vi "IECal-Create Queue Data.vi"(0 "state":T5, 7 "Params":T4) -> (8 "queue data":T1, 15 "error out":errorcluster)   [LabVIEW 2020]
uses:
  Typedefs/IECal-State.ctl
  Common VIs/Typedefs/CAL-Endpoint.ctl
  Typedefs/IECal-Parameters.ctl
  Common VIs/Typedefs/CAL-Stimulus.ctl
  Typedefs/IECal-Queue Data.ctl
  Typedefs/IECal-Response.ctl
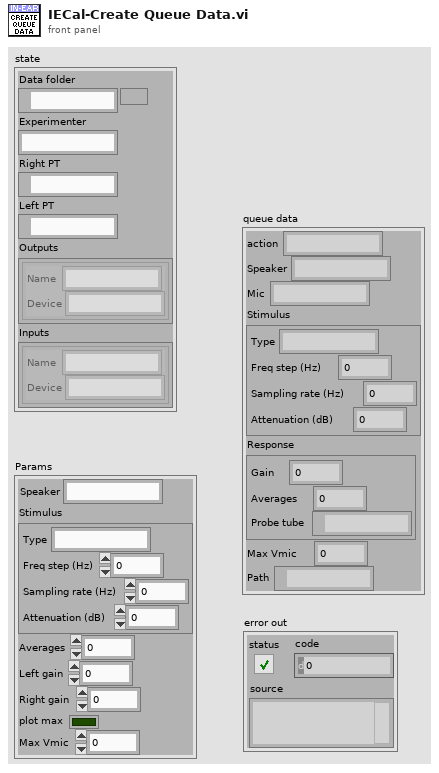
[diagram p1: front panel]
types:
  T1 = typedef "IECal-Queue Data.ctl" = cluster{"action":string, "Speaker":string, "Mic":string, "Stimulus":T2, "Response":T3, "Max Vmic":dbl, "Path":path}
  T2 = typedef "CAL-Stimulus.ctl" = cluster{"Type":string, "Freq step (Hz)":dbl, "Sampling rate (Hz)":dbl, "Attenuation (dB)":dbl}
  T3 = typedef "IECal-Response.ctl" = cluster{"Gain":dbl, "Averages":i32, "Probe tube":path}
  T4 = typedef "IECal-Parameters.ctl" = cluster{"Speaker":string, "Stimulus":T2, "Averages":i32, "Left gain":dbl, "Right gain":dbl, "plot max":bool, "Max Vmic":dbl}
  T5 = typedef "IECal-State.ctl" = cluster{"Data folder":path, "Experimenter":string, "Right PT":path, "Left PT":path, "Outputs":T6[], "Inputs":T6[]}
  T6 = typedef "CAL-Endpoint.ctl" = cluster{"Name":string, "Device":string}
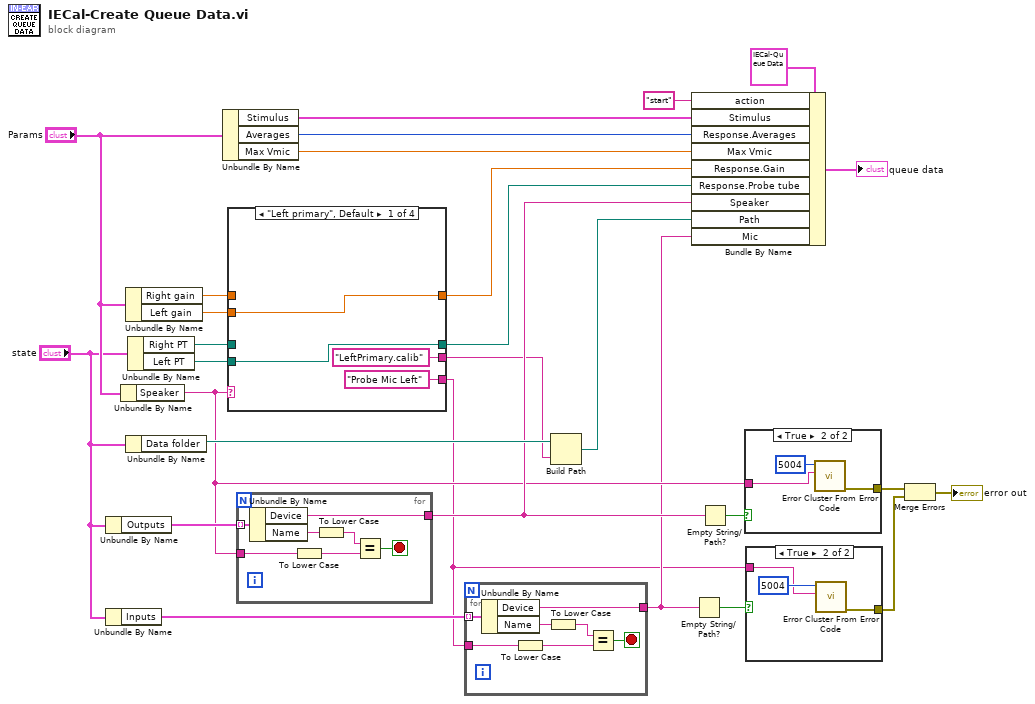
[diagram p0: block diagram]
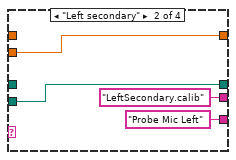
[diagram p4: hidden frame]
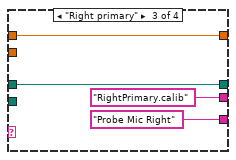
[diagram p5: hidden frame]
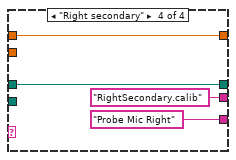
[diagram p6: hidden frame]
diagram:
  n1 = Unbundle By Name("state") -> ("Outputs"=w14:T6[])
  n2 = Unbundle By Name("state") -> ("Inputs"=w12:T6[])
  n3 = Unbundle By Name("Params") -> ("Speaker"=w9:string)
  n4 = Unbundle By Name("Params") -> ("Right gain"=w28:dbl, "Left gain"=w27:dbl)
  n5 = Unbundle By Name("state") -> ("Data folder"=w22:path)
  n6 = Unbundle By Name("state") -> ("Right PT"=w24:path, "Left PT"=w23:path)
  n7 = Unbundle By Name("Params") -> ("Stimulus"=w21:T2, "Averages"=w19:i32, "Max Vmic"=w17:dbl)
  n8 = case shown="\"Left primary\", Default" w9 {
    tunnel: w28 -> [_ _ w40 w44]
    tunnel: w27 -> [w32 w36 _ _]
    tunnel: [w32 w36 w40 w44] -> w16
    tunnel: w24 -> [_ _ w39 w43]
    tunnel: w23 -> [w31 w35 _ _]
    tunnel: [w31 w35 w39 w43] -> w15
    tunnel: ["Probe Mic Left" "Probe Mic Left" "Probe Mic Right" "Probe Mic Right"] -> w6
    tunnel: ["LeftPrimary.calib" "LeftSecondary.calib" "RightPrimary.calib" "RightSecondary.calib"] -> w2
    frame "Left primary", Default {
    }
    frame "Left secondary" {
    }
    frame "Right primary" {
    }
    frame "Right secondary" {
    }
  }
  n9 = for {
    tunnel: w14 -> [w51] mode=indexing
    tunnel: [w48] -> w11
    tunnel: w9 -> [w47]
    stop <- w49 stop-if-true
    n10 = Unbundle By Name(w51) -> ("Device"=w48:string, "Name"=w50:string)
    n11 = To Lower Case(string=w47) -> (all lower case string=w45:string)
    n12 = To Lower Case(string=w50) -> (all lower case string=w46:string)
    n13 = Equal?(x=w46, y=w45) -> (x = y?=w49:bool)
  }
  n14 = for {
    tunnel: w12 -> [w58] mode=indexing
    tunnel: [w55] -> w8
    tunnel: w6 -> [w54]
    stop <- w56 stop-if-true
    n15 = Unbundle By Name(w58) -> ("Device"=w55:string, "Name"=w57:string)
    n16 = To Lower Case(string=w54) -> (all lower case string=w52:string)
    n17 = To Lower Case(string=w57) -> (all lower case string=w53:string)
    n18 = Equal?(x=w53, y=w52) -> (x = y?=w56:bool)
  }
  n19 = Build Path(base path=w22, name or relative path=w2) -> (appended path=w1:path)
  n20 = Bundle By Name(cluster=T1 {"action"="", "Speaker"="", "Mic"="", "Stimulus"={"Type"="", "Freq step (Hz)"=0.0, "Sampling rate (Hz)"=0.0, "Attenuation (dB)"=0.0}, "Response"={"Gain"=0.0, "Averages"=0, "Probe tube"=path ""}, "Max Vmic"=0.0, "Path"=path ""} ("queue data"), "action"="start", "Stimulus"=w21, "Response.Averages"=w19, "Max Vmic"=w17, "Response.Gain"=w16, "Response.Probe tube"=w15, "Speaker"=w11, "Path"=w1, "Mic"=w8) -> (→"queue data":T1)
  n21 = Empty String/Path?(string/path=w8) -> (empty?=w7:bool)
  n22 = Empty String/Path?(string/path=w11) -> (empty?=w10:bool)
  n23 = case shown="True" w10 {
    tunnel: w9 -> [_ w60]
    tunnel: [_ w59] -> w5
    frame False {
    }
    frame True {
      n24 = call <vilib>:"Error Cluster From Error Code.vi"("error message (\"\")"=w60, "error code (0)"=5004) -> ("error out"=w59:errorcluster)  [unwired: 7 in]
    }
  }
  n25 = case shown="True" w7 {
    tunnel: [_ w63] -> w4
    tunnel: w6 -> [_ w62]
    frame False {
    }
    frame True {
      n26 = call <vilib>:"Error Cluster From Error Code.vi"("error message (\"\")"=w62, "error code (0)"=5004) -> ("error out"=w63:errorcluster)  [unwired: 7 in]
    }
  }
  n27 = Merge Errors(w5, w4) -> (→"error out":errorcluster)
